vi "Teleop.vi"(10 "Match Info":T2={"Autonomous Elapsed Seconds"=0.0, "TeleOp Elapsed Seconds"=0.0, "Disabled Elapsed Seconds"=0.0, "Visited Autonomous"=FALSE, "Visited TeleOp"=FALSE, "Visited Disabled"=FALSE, "Autonomous Settings"={"Autonomous Style"=enum."Independent", "VI Refnum"=refnum}}, 11 "Call Context":T3) -> ()   [LabVIEW 2015]
doc: "This VI is called for each TeleOp packet received from the DS where the robot is not disabled. It is often used to read from the joysticks and update I/O or to update setpoints for timed control loops. It should complete and return within 20 milliseconds or it may miss DS packets."
uses:
  <vilib>/Rock Robotics/WPI/DriverStation/WPI_DriverStationDerivedRobotMode.ctl
  <vilib>/Rock Robotics/WPI/DriverStation/WPI_DriverStationMatch Info.ctl
  <vilib>/Rock Robotics/SystemInterfaces/spilib/spi_bus.ctl
  <vilib>/Rock Robotics/WPI/CAN/TalonSRX/WPI_CANTalonSRX_APIFeedbackSelect.ctl
  <vilib>/Rock Robotics/WPI/CAN/TalonSRX/WPI_CANTalonSRX_APIControlMode.ctl
  <vilib>/Rock Robotics/WPI/Utilities/WPI_GetSetVariantRefNum.vi
  <vilib>/Rock Robotics/Network Tables/NT Write Boolean Array.vi
  <vilib>/Rock Robotics/Network Tables/NT Write Numeric Array.vi
  <vilib>/Rock Robotics/Network Tables/NT Read Boolean.vi
  <vilib>/Rock Robotics/Network Tables/NT Read Number.vi
  <vilib>/Rock Robotics/WPI/RobotDrive/WPI_RobotDriveArcadeDrive_Standard(NoSaturation).vi
  <vilib>/Rock Robotics/WPI/CAN/Jaguar/SubVIs/WPI_CANJaguar_ControlMode.ctl
  Program Files/National Instruments/LabVIEW 2016/LabVIEW 2016/Targets/NI/RT/VxWorks/vi.lib/Rock Robotics/WPI/CAN/Jaguar/SubVIs/WPI_CANJaguar_SpeedReference.ctl
  <vilib>/Rock Robotics/WPI/Gyro/WPI_GyroAnalogOpen.vi
  <vilib>/Rock Robotics/WPI/MotorControl/WPI_MotorControlOpenCANTalonSRX.vi
  <vilib>/Rock Robotics/Network Tables/NT Write Number.vi
  <vilib>/Rock Robotics/WPI/MotorControl/WPI_MotorControlOpenCANJaguar.vi
panel:
  out "Device Found":bool
  in  "SPI Bus":T1
  in  "Sample Rate (ms)":dbl=1.0 min=0.0 max=100.0 step=0.25 format="%#_13g"
  out "Angle":dbl(knob) scale=0.0..360.0
  in  "stop 2":bool
  in  "Reset Angle?":bool
  out "Calibrated?":bool
  out "Sample Slider 0":dbl(slide) scale=0.0..5.0
  out "Sample Boolean 1":bool
  out "Sample Boolean 0":bool
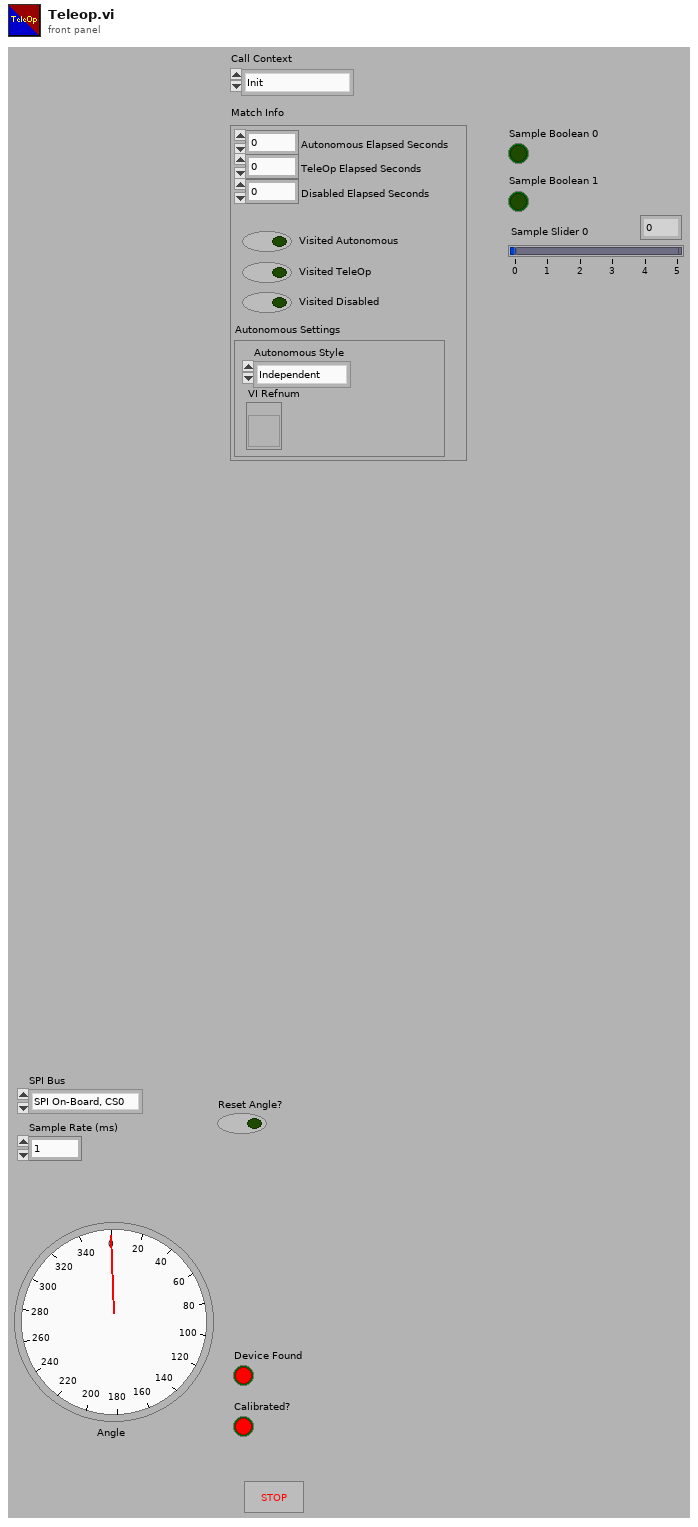
[diagram p1: front panel]
types:
  T1 = typedef "spi_bus.ctl" = enum16{"SPI On-Board, CS0", "SPI On-Board, CS1", "SPI On-Board, CS2", "SPI On-Board, CS3", "SPI MXP", "Invalid"}
  T2 = typedef "WPI_DriverStationMatch Info.ctl" = cluster{"Autonomous Elapsed Seconds":dbl, "TeleOp Elapsed Seconds":dbl, "Disabled Elapsed Seconds":dbl, "Visited Autonomous":bool, "Visited TeleOp":bool, "Visited Disabled":bool, "Autonomous Settings":cluster{"Autonomous Style":enum16{"Iterative", "Independent"}, "VI Refnum":refnum<vi>}}
  T3 = typedef "WPI_DriverStationDerivedRobotMode.ctl" = enum16{"Init", "Execute", "Stop"}
  T4 = typedef "WPI_JoystickDevRef.ctl" = cluster{"Device":T5}
  T5 = typedef "WPI_JoystickDeviceEnum.ctl" = enum16{"USB 0", "USB 1", "USB 2", "USB 3", "USB 4", "USB 5"}
  T6 = cluster{"Axes[0]":dbl, "Axes[1]":dbl, "Axes[2]":dbl, "Axes[3]":dbl, "Axes[4]":dbl, "Axes[5]":dbl, "Axes[6]":dbl, "Axes[7]":dbl, "Axes[8]":dbl}
  T7 = cluster{"Buttons[0]":bool, "Buttons[1]":bool, "Buttons[2]":bool, "Buttons[3]":bool, "Buttons[4]":bool, "Buttons[5]":bool, "Buttons[6]":bool, "Buttons[7]":bool, "Buttons[8]":bool}
  T8 = typedef "WPI_MotorControlDeviceRef.ctl" = cluster{"DeviceStatus":errorcluster, "Type":T9, "PWM":cluster{"PWM Channel":T10, "DeadBand":T11}, "CAN":cluster{"Device Number":u8, "Control Mode":T12, "Semaphore":T13, "Max Vout":dbl, "TalonSRX Control Mode":T14}, "Invert":bool}
  T9 = typedef "WPI_MotorControlType.ctl" = enum16{"PWM", "CAN", "CANTalonSRX"}
  T10 = typedef "FPGA_DIOPWMChannel.ctl" = enum8{"PWM 0", "PWM 1", "PWM 2", "PWM 3", "PWM 4", "PWM 5", "PWM 6", "PWM 7", "PWM 8", "PWM 9", "PWM MXP 0", "PWM MXP 1", "PWM MXP 2", "PWM MXP 3", "PWM MXP 4", "PWM MXP 5", "PWM MXP 6", "PWM MXP 7", "PWM MXP 8", "PWM MXP 9", "Invalid"}
  T11 = typedef "WPI_PWMDeadband.ctl" = cluster{"Name":string, "maxPositivePwm":i32, "minPositivePwm":i32, "centerPwm":i32, "maxNegativePwm":i32, "minNegativePwm":i32, "angularRange":u16}
  T12 = typedef "WPI_CANJaguar_ControlMode.ctl" = enum8{"Percent VBus", "Current", "Speed", "Position", "Voltage"}
  T13 = typedef "Semaphore RefNum" = refnum<k1>
  T14 = typedef "WPI_CANTalonSRX_APIControlMode.ctl" = enum8{"Percent VBus", "Speed", "Position", "Slave", "Unchanged / Invalid", "Voltage Compensation", "Current", "Motion Profile"}
  T15 = typedef "WPI_RobotDriveDevRef.ctl" = cluster{"DevStatus":errorcluster, "Motors[]":T8[], "Square Inputs":bool, "Max Output":dbl}
  T16 = typedef "WPI_SwitchDevRef.ctl" = cluster{"DevStatus":errorcluster, "DIO Channel":T17, "CntIndex":T18, "Normally Closed":bool}
  T17 = typedef "FPGA_DIOChannel.ctl" = enum8{"DIO 0", "DIO 1", "DIO 2", "DIO 3", "DIO 4", "DIO 5", "DIO 6", "DIO 7", "DIO 8", "DIO 9", "DIO MXP 0", "DIO MXP 1", "DIO MXP 2", "DIO MXP 3", "DIO MXP 4", "DIO MXP 5", "DIO MXP 6", "DIO MXP 7", "DIO MXP 8", "DIO MXP 9", "DIO MXP 10", "DIO MXP 11", "DIO MXP 12", "DIO MXP 13", "DIO MXP 14", "DIO MXP 15", "Invalid"}
  T18 = typedef "FPGA_CounterCtrSystemIndex.ctl" = enum8{"Ctr 0", "Ctr 1", "Ctr 2", "Ctr 3", "Ctr 4", "Ctr 5", "Ctr 6", "Ctr 7", "Invalid"}
  T19 = typedef "WPI_GyroDevRef.ctl" = cluster{"DevStatus":errorcluster, "Analog Channel":T20, "Offset":dbl, "Gain (VoltsPerDegree/Second)":dbl, "Gyro Type":enum16{"Analog", "XRS450"}, "Handle":i32, "SPI Bus":T1, "Device Found":bool, "Sample Rate":dbl, "Calibrate On Open":bool}
  T20 = typedef "FPGA_AIChannel.ctl" = enum8{"AI 0", "AI 1", "AI 2", "AI 3", "AI MXP 0", "AI MXP 1", "AI MXP 2", "AI MXP 3", "Invalid"}
  T21 = typedef "WPI_CANTalonSRX_APIFeedbackSelect.ctl" = enum16{"Digital Quadrature Encoder", "Analog Potentiometer", "Analog Encoder", "Count on Quad-A (Rising-Edge)", "Count on Quad-A (Falling-Edge)", "CTR Magnetic Enc (Absolute)", "CTR Magnetic Enc (Relative)", "Pulse Width"}
  T22 = typedef "WPI_CANJaguar_SpeedReference.ctl" = u8
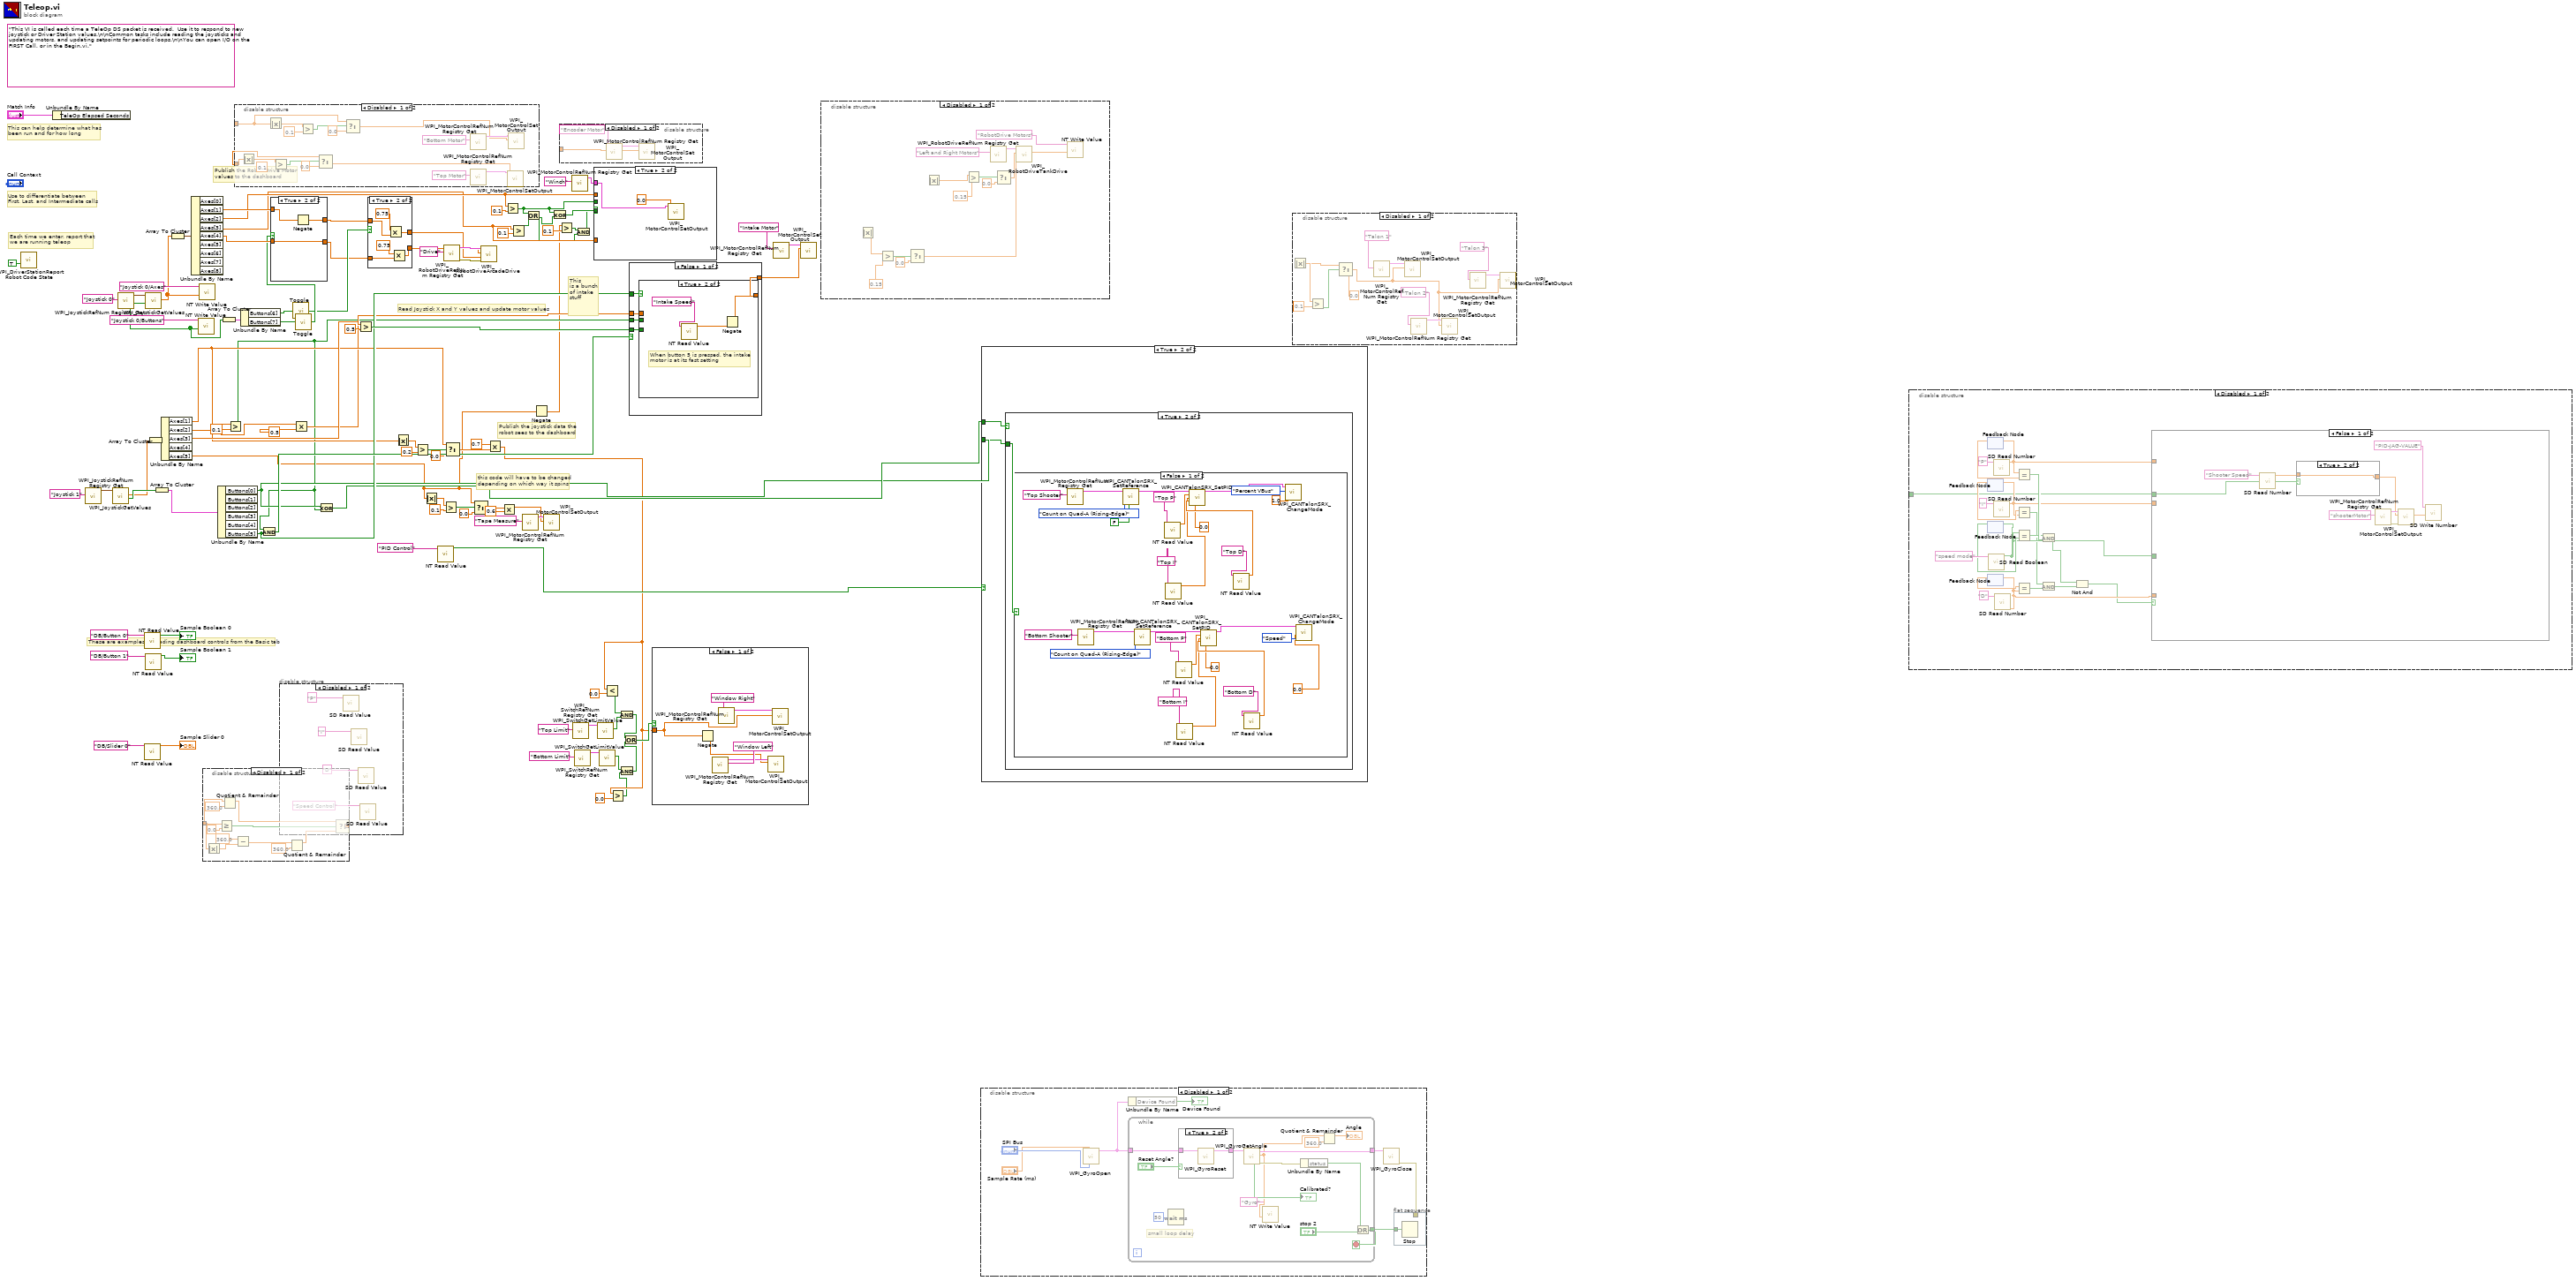
[diagram p0: block diagram]
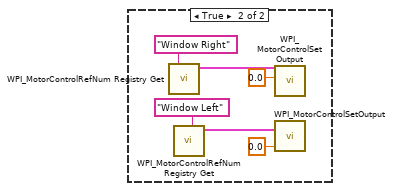
[diagram p2: hidden frame]
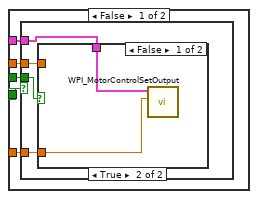
[diagram p3: hidden frame]
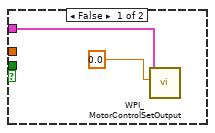
[diagram p4: hidden frame]
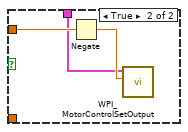
[diagram p5: hidden frame]
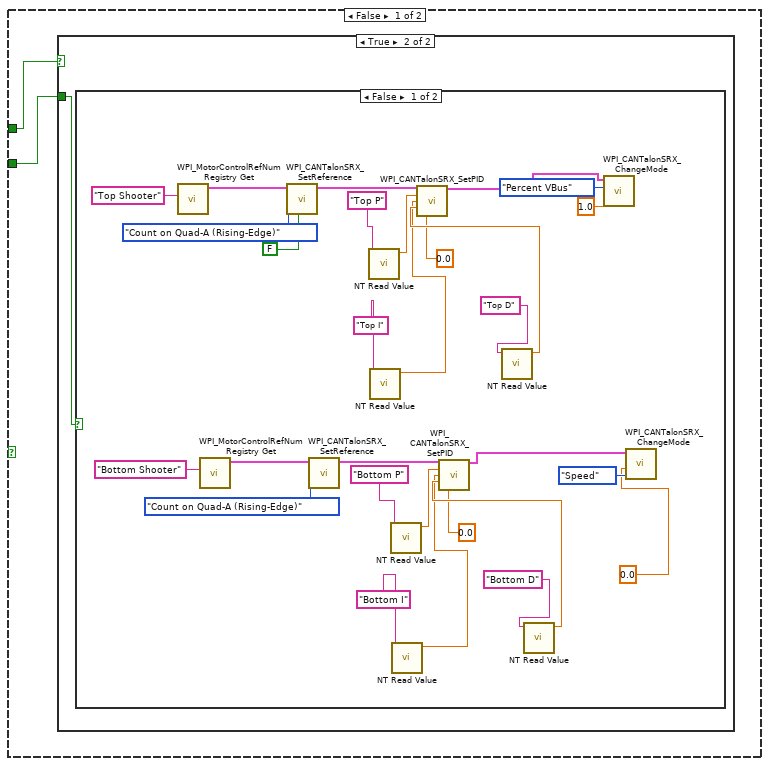
[diagram p6: hidden frame]
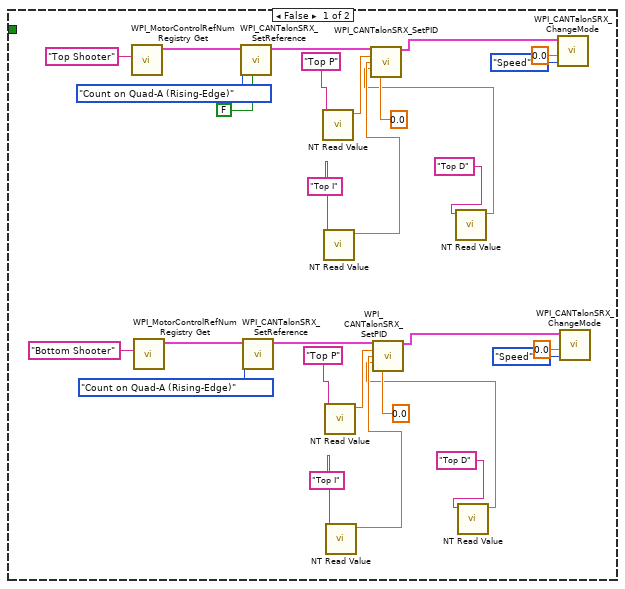
[diagram p7: hidden frame]
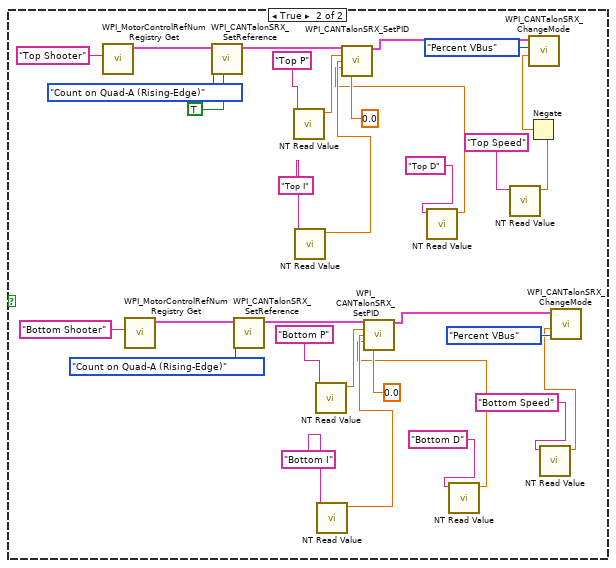
[diagram p8: hidden frame]
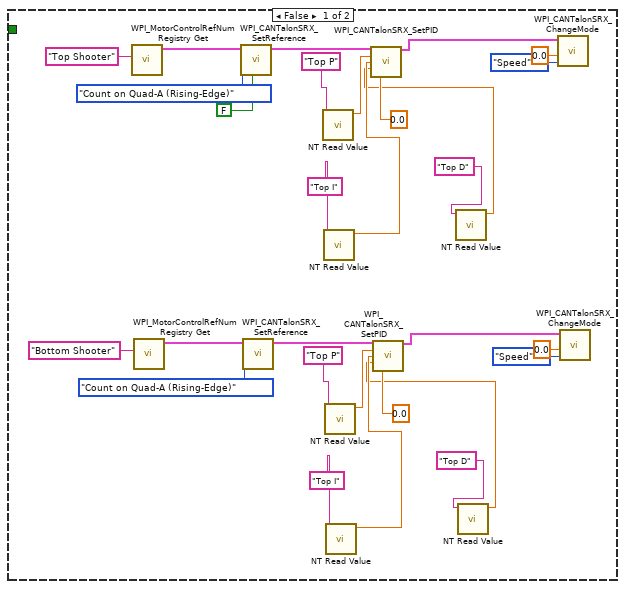
[diagram p9: hidden frame]
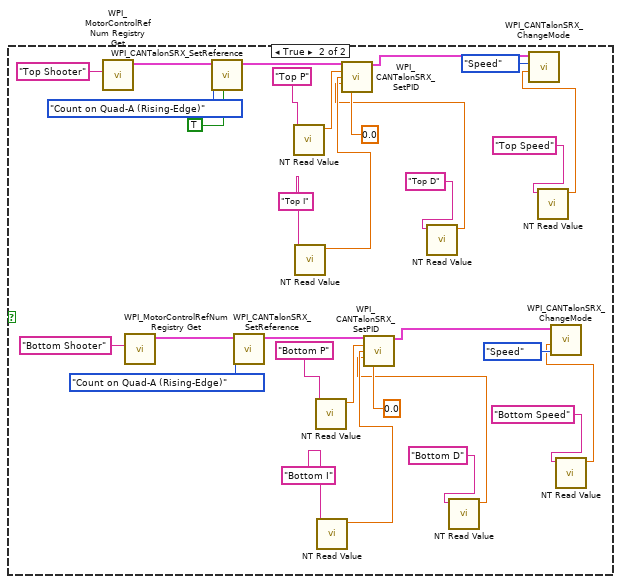
[diagram p10: hidden frame]
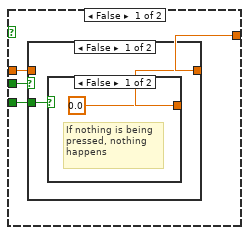
[diagram p14: hidden frame]
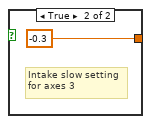
[diagram p15: hidden frame]
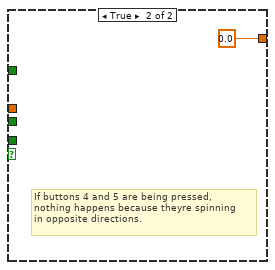
[diagram p17: hidden frame]
diagram:
  (unwired) "This VI is called each time a TeleOp DS packet is received.  Use it to respond to new joystick or Driver Station values.\n\nCommon tasks include reading the joysticks and updating motors, and updating setpoints for periodic loops.\n\nYou can open I/O on the FIRST Call, or in the Begin.vi."
  # "this code will have to be changed\ndepending on which way it spins"
  # "This \nis a bunch\nof intake\nstuff"
  # "These are examples of reading dashboard controls from the Basic tab"
  # "Publish the Robot Drive Motor\nvalues to the dashboard"
  # "Publish the joystick data the\nrobot sees to the dashboard"
  # "Each time we enter, report that\nwe are running teleop"
  # "Use to differentiate between\nFirst, Last, and Intermediate calls"
  # "This can help determine what has\nbeen run and for how long"
  # "Read Joystick X and Y values and update motor values"
  n1 = call <vilib>:"WPI_DriverStationReport Robot Code State.vi"("TeleOp"=TRUE ("Autonomous")) -> ()  [unwired: 10 in, 1 out]
  n2 = Unbundle By Name("Match Info") -> ()  [unwired: 1 out]
  n3 = call <vilib>:"WPI_JoystickRefNum Registry Get.vi"("refnum name"="Joystick 1") -> ("JoystickDevRef"=w75:T4)  [unwired: 1 in, 9 out]
  n4 = call <vilib>:"WPI_JoystickGetValues.vi"("JoystickDevRef"=w75) -> ("Buttons"=w74:bool[], "Axes"=w72:dbl[])  [unwired: 6 in, 3 out]
  n5 = call <vilib>:"WPI_JoystickRefNum Registry Get.vi"("refnum name"="Joystick 0") -> ("JoystickDevRef"=w95:T4)  [unwired: 1 in, 9 out]
  n6 = call-poly <vilib>:"NT Read Value.vi"("Name"="DB/Button 0" ("refnum name")) -> ("Boolean"=→"Sample Boolean 0":bool)  [unwired: 9 in, 1 out]
  n7 = call-poly <vilib>:"NT Read Value.vi"("Name"="DB/Slider 0" ("refnum name")) -> ("Numeric"=→"Sample Slider 0":dbl)  [unwired: 9 in, 1 out]
  n8 = call-poly <vilib>:"NT Read Value.vi"("Name"="DB/Button 1" ("refnum name")) -> ("Boolean"=→"Sample Boolean 1":bool)  [unwired: 9 in, 1 out]
  n9 = call <vilib>:"WPI_JoystickGetValues.vi"("JoystickDevRef"=w95) -> ("Buttons"=w69:bool[], "Axes"=w85:dbl[])  [unwired: 6 in, 3 out]
  n10 = Array To Cluster(array=w72) -> (cluster=w71:T6)
  n11 = Array To Cluster(array=w74) -> (cluster=w73:T7)
  n12 = Unbundle By Name(w71) -> ("Axes[1]"=w56:dbl, "Axes[2]"=w45:dbl, "Axes[3]"=w70:dbl, "Axes[5]"=w27:dbl)  [unwired: 1 out]
  n13 = Array To Cluster(array=w85) -> (cluster=w84:T6)
  n14 = Unbundle By Name(w84) -> ("Axes[1]"=w62:dbl, "Axes[2]"=w30:dbl, "Axes[3]"=w29:dbl, "Axes[4]"=w63:dbl)  [unwired: 5 out]
  n15 = call-poly <vilib>:"NT Write Value.vi"("Boolean Array"=w69, "Name"="Joystick 0/Buttons") -> ()  [unwired: 9 in, 1 out]
  n16 = call-poly <vilib>:"NT Write Value.vi"("Numeric Array"=w85, "Name"="Joystick 0/Axes") -> ()  [unwired: 9 in, 1 out]
  n17 = disable-structure shown="Disabled" {
    disable-tunnel: _ -> [w103 _]
    disable-tunnel: [w98 _] -> _
    frame Disabled {
      n18 = Absolute Value(x=w103) -> (abs(x)=w102:dbl)
      n19 = Greater Or Equal?(x=w103, y=0.0) -> (x >= y?=w106:bool)
      n20 = Quotient & Remainder(x=w103, y=360.0) -> (x-y*floor(x/y)=w105:dbl)  [unwired: 1 out]
      n21 = Subtract(x=360.0, y=w102) -> (x-y=w101:dbl)
      n22 = Quotient & Remainder(x=w101, y=360.0) -> (x-y*floor(x/y)=w99:dbl)  [unwired: 1 out]
      n23 = Select(t=w105, s=w106, f=w99) -> (s? t:f=w98:dbl)
    }
    frame Enabled {
    }
  }
  n24 = Unbundle By Name(w73) -> ("Buttons[0]"=w35:bool, "Buttons[5]"=w77:bool)  [unwired: 4 out]
  n25 = Array To Cluster(array=w69) -> (cluster=w68:T7)
  n26 = Greater?(x=w45, y=0.1) -> (0:w34:bool)
  n27 = disable-structure shown="Disabled" {
    disable-tunnel: _ -> [w116 _]
    disable-tunnel: _ -> [w109 _]
    frame Disabled {
      n28 = Absolute Value(x=w116) -> (abs(x)=w119:dbl)
      n29 = Absolute Value(x=w109) -> (abs(x)=w114:dbl)
      n30 = Greater?(x=w119, y=0.1) -> (0:w117:bool)
      n31 = Greater?(x=w114, y=0.1) -> (0:w112:bool)
      n32 = Select(t=w116, s=w117, f=0.0) -> (s? t:f=w120:dbl)
      n33 = Select(t=w109, s=w112, f=0.0) -> (s? t:f=w110:dbl)
      n34 = call <vilib>:"WPI_MotorControlRefNum Registry Get.vi"("refnum name"="Bottom Motor") -> ("MotorControlDevRef"=w121:T8)  [unwired: 9 in, 1 out]
      n35 = call <vilib>:"WPI_MotorControlRefNum Registry Get.vi"("refnum name"="Top Motor") -> ("MotorControlDevRef"=w122:T8)  [unwired: 9 in, 1 out]
      n36 = call <vilib>:"WPI_MotorControlSetOutput.vi"("Output"=w120, "MotorControlDevRef"=w122) -> ()  [unwired: 7 in, 3 out]
      n37 = call <vilib>:"WPI_MotorControlSetOutput.vi"("Output"=w110, "MotorControlDevRef"=w121) -> ()  [unwired: 7 in, 3 out]
    }
    frame Enabled {
    }
  }
  n38 = Unbundle By Name(w68) -> ("Buttons[6]"=w53:bool, "Buttons[7]"=w67:bool)
  n39 = And(x=w34, y=w77) -> (x .and. y?=w81:bool)
  n40 = disable-structure shown="Disabled" {
    frame Disabled {
      n41 = call-poly <vilib>:"SD Read Value.vi"("Name"="P") -> ()  [unwired: 8 in, 3 out]
      n42 = call-poly <vilib>:"SD Read Value.vi"("Name"="I") -> ()  [unwired: 8 in, 3 out]
      n43 = call-poly <vilib>:"SD Read Value.vi"("Name"="D") -> ()  [unwired: 8 in, 3 out]
      n44 = call-poly <vilib>:"SD Read Value.vi"("Name"="Speed Control") -> ()  [unwired: 8 in, 3 out]
    }
    frame Enabled {
    }
  }
  n45 = call "Toggle.vi"("Input"=w53) -> ("Output"=w52:bool)
  n46 = Multiply(x=w45, y=0.5) -> (x*y=w47:dbl)
  n47 = call "Toggle.vi"("Input"=w67) -> ("Output"=w61:bool)
  n48 = case shown="True" w61 {
    tunnel: [w129 w133] -> w51
    tunnel: w63 -> [w129 w133]
    tunnel: [w130 w131] -> w50
    tunnel: w62 -> [w130 w132]
    frame False {
    }
    frame True {
      n49 = Negate(x=w132) -> (-x=w131:dbl)
    }
  }
  n50 = Exclusive Or(1:w34, 2:w35) -> (0:w36:bool)
  n51 = Greater?(x=w70, y=0.5) -> (0:w79:bool)
  n52 = case shown="True" w52 {
    tunnel: w51 -> [w134 w139]
    tunnel: w50 -> [w135 w138]
    tunnel: [w135 w137] -> w49
    tunnel: [w134 w136] -> w48
    frame False {
    }
    frame True {
      n53 = Multiply(x=0.75, y=w138) -> (x*y=w137:dbl)
      n54 = Multiply(x=0.75, y=w139) -> (x*y=w136:dbl)
    }
  }
  n55 = Absolute Value(x=w56) -> (abs(x)=w57:dbl)
  n56 = Greater?(x=w57, y=0.2) -> (0:w59:bool)
  n57 = Absolute Value(x=w27) -> (abs(x)=w41:dbl)
  n58 = call-poly <vilib>:"NT Read Value.vi"("Name"="PID Control") -> ("Boolean"=w15:bool)  [unwired: 9 in, 1 out]
  n59 = Greater?(x=w41, y=0.1) -> (0:w43:bool)
  n60 = call <vilib>:"WPI_RobotDriveRefNum Registry Get.vi"("refnum name"="Drive") -> ("error out"=w64:errorcluster, "RobotDriveDevRef"=w65:T15)  [unwired: 1 in, 8 out]
  n61 = Select(t=w56, s=w59, f=0.0) -> (s? t:f=w60:dbl)
  n62 = Select(t=w27, s=w43, f=0.0) -> (s? t:f=w37:dbl)
  n63 = call-poly <vilib>:"WPI_RobotDriveArcadeDrive.vi"("error in (no error)"=w64, "Y axis value"=w49, "X axis value"=w48, "RobotDriveDevRef"=w65) -> ()  [unwired: 5 in, 3 out]
  n64 = Multiply(x=0.7, y=w60) -> (x*y=w7:dbl)
  n65 = Multiply(x=w37, y=0.6) -> (x*y=w22:dbl)
  n66 = Greater?(x=w30, y=0.1) -> (0:w25:bool)
  n67 = Greater?(x=w29, y=0.1) -> (0:w24:bool)
  n68 = call <vilib>:"WPI_MotorControlRefNum Registry Get.vi"("refnum name"="Tape Measure") -> ("MotorControlDevRef"=w39:T8)  [unwired: 9 in, 1 out]
  n69 = Or(x=w25, y=w24) -> (x .or. y?=w23:bool)
  n70 = Negate(x=w27) -> (-x=w17:dbl)
  n71 = call <vilib>:"WPI_MotorControlSetOutput.vi"("Output"=w22, "MotorControlDevRef"=w39) -> ()  [unwired: 7 in, 3 out]
  n72 = Exclusive Or(1:w24, 2:w25) -> (0:w31:bool)
  n73 = Greater?(x=w17, y=0.1) -> (0:w26:bool)
  n74 = disable-structure shown="Disabled" {
    disable-tunnel: _ -> [w142 _]
    frame Disabled {
      n75 = call <vilib>:"WPI_MotorControlRefNum Registry Get.vi"("refnum name"="Encoder Motor") -> ("MotorControlDevRef"=w143:T8)  [unwired: 9 in, 1 out]
      n76 = call <vilib>:"WPI_MotorControlSetOutput.vi"("Output"=w142, "MotorControlDevRef"=w143) -> ()  [unwired: 7 in, 3 out]
    }
    frame Enabled {
    }
  }
  n77 = call <vilib>:"WPI_MotorControlRefNum Registry Get.vi"("refnum name"="Winch") -> ("MotorControlDevRef"=w18:T8)  [unwired: 9 in, 1 out]
  n78 = call <vilib>:"WPI_SwitchRefNum Registry Get.vi"("refnum name"="Top Limit") -> ("SwitchDevRef"=w14:T16)  [unwired: 9 in, 1 out]
  n79 = call <vilib>:"WPI_SwitchRefNum Registry Get.vi"("refnum name"="Bottom Limit") -> ("SwitchDevRef"=w12:T16)  [unwired: 9 in, 1 out]
  n80 = And(x=w26, y=w23) -> (x .and. y?=w20:bool)
  n81 = case shown="True" w20 {
    tunnel: w31 -> [w149 _]
    tunnel: w30 -> [w148 _]
    tunnel: w29 -> [w147 _]
    tunnel: w25 -> [w146 _]
    tunnel: w18 -> [w145 w161]
    frame False {
      n82 = case shown="True" w149 {
        tunnel: w146 -> [_ w155]
        tunnel: w148 -> [_ w154]
        tunnel: w147 -> [_ w153]
        tunnel: w145 -> [w150 w152]
        frame False {
          n83 = call <vilib>:"WPI_MotorControlSetOutput.vi"("Output"=0.0, "MotorControlDevRef"=w150) -> ()  [unwired: 7 in, 3 out]
        }
        frame True {
          n84 = case shown="False" w155 {
            tunnel: w154 -> [_ w160]
            tunnel: w153 -> [w157 _]
            tunnel: w152 -> [w156 w158]
            frame False {
              n85 = call <vilib>:"WPI_MotorControlSetOutput.vi"("Output"=w157, "MotorControlDevRef"=w156) -> ()  [unwired: 7 in, 3 out]
            }
            frame True {
              n86 = Negate(x=w160) -> (-x=w159:dbl)
              n87 = call <vilib>:"WPI_MotorControlSetOutput.vi"("Output"=w159, "MotorControlDevRef"=w158) -> ()  [unwired: 7 in, 3 out]
            }
          }
        }
      }
    }
    frame True {
      n88 = call <vilib>:"WPI_MotorControlSetOutput.vi"("Output"=0.0, "MotorControlDevRef"=w161) -> ()  [unwired: 7 in, 3 out]
    }
  }
  n89 = call <vilib>:"WPI_SwitchGetLimitValue.vi"("SwitchDevRef"=w14) -> ("Switch Pressed"=w1:bool)  [unwired: 8 in, 2 out]
  n90 = call <vilib>:"WPI_SwitchGetLimitValue.vi"("SwitchDevRef"=w12) -> ("Switch Pressed"=w5:bool)  [unwired: 8 in, 2 out]
  n91 = Less?(x=w7, y=0.0) -> (x < y?=w8:bool)
  n92 = Greater?(x=w7, y=0.0) -> (0:w4:bool)
  n93 = And(x=w8, y=w1) -> (x .and. y?=w2:bool)
  n94 = And(x=w5, y=w4) -> (x .and. y?=w3:bool)
  n95 = Or(x=w2, y=w3) -> (x .or. y?=w10:bool)
  n96 = case shown="False" w81 {
    tunnel: [w166 0.0] -> w78
    tunnel: w77 -> [w167 _]
    tunnel: w79 -> [w165 _]
    tunnel: w47 -> [w164 _]
    tunnel: w34 -> [w163 _]
    frame False {
      n97 = case shown="True" w167 {
        tunnel: [w171 w177] -> w166
        tunnel: w165 -> [w170 _]
        tunnel: w164 -> [w169 _]
        tunnel: w163 -> [w168 _]
        frame False {
          n98 = case shown="False" w168 {
            tunnel: [w172 w176] -> w171
            tunnel: w170 -> [w173 _]
            tunnel: w169 -> [_ w176]
            frame False {
              n99 = case shown="False" w173 {
                tunnel: [0.0 -0.3] -> w172
                frame False {
                  # "If nothing is being\npressed, nothing \nhappens"
                }
                frame True {
                  # "Intake slow setting\nfor axes 3"
                }
              }
            }
            frame True {
              # "When button\n4 is being pressed,\nthe outake is activated"
            }
          }
        }
        frame True {
          # "When button 5 is pressed, the intake \nmotor is at its fast setting"
          n100 = call-poly <vilib>:"NT Read Value.vi"("Name"="Intake Speed") -> ("Numeric"=w178:dbl)  [unwired: 9 in, 1 out]
          n101 = Negate(x=w178) -> (-x=w177:dbl)
        }
      }
    }
    frame True {
      # "If buttons 4 and 5 are being pressed,\nnothing happens because theyre spinning\nin opposite directions."
    }
  }
  n102 = case shown="False" w10 {
    tunnel: w7 -> [w181 _]
    frame False {
      n103 = Negate(x=w181) -> (-x=w182:dbl)
      n104 = call <vilib>:"WPI_MotorControlRefNum Registry Get.vi"("refnum name"="Window Left") -> ("MotorControlDevRef"=w185:T8)  [unwired: 9 in, 1 out]
      n105 = call <vilib>:"WPI_MotorControlRefNum Registry Get.vi"("refnum name"="Window Right") -> ("MotorControlDevRef"=w184:T8)  [unwired: 9 in, 1 out]
      n106 = call <vilib>:"WPI_MotorControlSetOutput.vi"("Output"=w182, "MotorControlDevRef"=w185) -> ()  [unwired: 7 in, 3 out]
      n107 = call <vilib>:"WPI_MotorControlSetOutput.vi"("Output"=w181, "MotorControlDevRef"=w184) -> ()  [unwired: 7 in, 3 out]
    }
    frame True {
      n108 = call <vilib>:"WPI_MotorControlRefNum Registry Get.vi"("refnum name"="Window Right") -> ("MotorControlDevRef"=w191:T8)  [unwired: 9 in, 1 out]
      n109 = call <vilib>:"WPI_MotorControlRefNum Registry Get.vi"("refnum name"="Window Left") -> ("MotorControlDevRef"=w190:T8)  [unwired: 9 in, 1 out]
      n110 = call <vilib>:"WPI_MotorControlSetOutput.vi"("Output"=0.0, "MotorControlDevRef"=w191) -> ()  [unwired: 7 in, 3 out]
      n111 = call <vilib>:"WPI_MotorControlSetOutput.vi"("Output"=0.0, "MotorControlDevRef"=w190) -> ()  [unwired: 7 in, 3 out]
    }
  }
  n112 = call <vilib>:"WPI_MotorControlRefNum Registry Get.vi"("refnum name"="Intake Motor") -> ("MotorControlDevRef"=w82:T8)  [unwired: 9 in, 1 out]
  n113 = call <vilib>:"WPI_MotorControlSetOutput.vi"("Output"=w78, "MotorControlDevRef"=w82) -> ()  [unwired: 7 in, 3 out]
  n114 = disable-structure shown="Disabled" {
    frame Disabled {
      n115 = Absolute Value() -> (abs(x)=w194:dbl)  [unwired: 1 in]
      n116 = Greater?(x=w194, y=0.15 ("x")) -> (0:w199:bool)
      n117 = Select(s=w199, f=0.0) -> (s? t:f=w197:dbl)  [unwired: 1 in]
      n118 = Absolute Value() -> (abs(x)=w193:dbl)  [unwired: 1 in]
      n119 = Greater?(x=w193, y=0.15 ("x")) -> (0:w202:bool)
      n120 = call <vilib>:"WPI_RobotDriveRefNum Registry Get.vi"("refnum name"="Left and Right Motors") -> ("RobotDriveDevRef"=w205:T15)  [unwired: 1 in, 9 out]
      n121 = Select(s=w202, f=0.0) -> (s? t:f=w200:dbl)  [unwired: 1 in]
      n122 = call <vilib>:"WPI_RobotDriveTankDrive.vi"("Right axis value"=w197, "Left axis value"=w200, "RobotDriveDevRef"=w205) -> ("Motor Values"=w204:dbl[])  [unwired: 6 in, 2 out]
      n123 = call-poly <vilib>:"NT Write Value.vi"("Numeric Array"=w204, "Name"="RobotDrive Motors") -> ()  [unwired: 9 in, 1 out]
    }
    frame Enabled {
    }
  }
  n124 = disable-structure shown="Disabled" {
    frame Disabled {
      n125 = call-poly <vilib>:"WPI_GyroOpen.vi"("Calibrated Center Voltage"="SPI Bus", "Calibration Time (s)"="Sample Rate (ms)") -> ("GyroDevRef"=w209:T19)  [unwired: 7 in, 2 out]
      n126 = Unbundle By Name(w209) -> ("Device Found"=→"Device Found":bool)
      n127 = while {
        tunnel: w209 -> [w224]
        tunnel: [w221] -> w211
        tunnel: [w219] -> w212
        stop <- w221 stop-if-true
        # "small loop delay"
        n128 = Wait (ms)(milliseconds to wait=u32 50) -> ()  [unwired: 1 out]
        n129 = case shown="True" "Reset Angle?" {
          tunnel: w224 -> [w229 w231]
          tunnel: [w229 w230] -> w220
          frame False {
          }
          frame True {
            n130 = call <vilib>:"WPI_GyroReset.vi"("GyroDevRef"=w231) -> ("GyroDevRef"=w230:T19)  [unwired: 9 in, 1 out]
          }
        }
        n131 = call <vilib>:"WPI_GyroGetAngle.vi"("GyroDevRef"=w220) -> ("error out"=w218:errorcluster, "Angle"=w216:dbl, "GyroDevRef"=w219:T19, "Calibrated?"=→"Calibrated?":bool)  [unwired: 6 in, 1 out]
        n132 = call-poly <vilib>:"NT Write Value.vi"("Numeric"=w216, "Name"="Gyro") -> ()  [unwired: 9 in, 1 out]
        n133 = Unbundle By Name(w218) -> ("status"=w222:bool)
        n134 = Quotient & Remainder(x=w216, y=360.0) -> (x-y*floor(x/y)=→"Angle":dbl)  [unwired: 1 out]
        n135 = Or(x=w222, y="stop 2") -> (x .or. y?=w221:bool)
      }
      n136 = call <vilib>:"WPI_GyroClose.vi"("GyroDevRef"=w212) -> ("error out"=w210:errorcluster)  [unwired: 10 in]
      n137 = flat-sequence {
        tunnel: w211 -> [w214]
        tunnel: w210 -> [_]
        frame #0 {
          n138 = Stop(stop? (T)=w214) -> ()
        }
      }
    }
    frame Enabled {
    }
  }
  n139 = case shown="True" w15 {
    tunnel: w36 -> [w233 w326]
    tunnel: w35 -> [w232 w325]
    frame False {
      n140 = case shown="True" w233 {
        tunnel: w232 -> [_ w263]
        frame False {
          n141 = call <vilib>:"WPI_MotorControlRefNum Registry Get.vi"("refnum name"="Top Shooter") -> ("MotorControlDevRef"=w261:T8)  [unwired: 9 in, 1 out]
          n142 = call <vilib>:"WPI_MotorControlRefNum Registry Get.vi"("refnum name"="Bottom Shooter") -> ("MotorControlDevRef"=w247:T8)  [unwired: 9 in, 1 out]
          n143 = call <vilib>:"WPI_CANTalonSRX_SetReference.vi"("Reverse Closed-Loop Output"=FALSE, "Feedback Reference"=WPI_CANTalonSRX_APIFeedbackSelect."Count on Quad-A (Rising-Edge)", "CAN Talon SRX Ref"=w261) -> ("CAN Talon SRX Ref"=w262:T8)  [unwired: 7 in, 1 out]
          n144 = call <vilib>:"WPI_CANTalonSRX_SetReference.vi"("Feedback Reference"=WPI_CANTalonSRX_APIFeedbackSelect."Count on Quad-A (Rising-Edge)", "CAN Talon SRX Ref"=w247) -> ("CAN Talon SRX Ref"=w248:T8)  [unwired: 8 in, 1 out]
          n145 = call-poly <vilib>:"NT Read Value.vi"("Name"="Top P") -> ("Numeric"=w252:dbl)  [unwired: 9 in, 1 out]
          n146 = call-poly <vilib>:"NT Read Value.vi"("Name"="Top I") -> ("Numeric"=w251:dbl)  [unwired: 9 in, 1 out]
          n147 = call-poly <vilib>:"NT Read Value.vi"("Name"="Top P") -> ("Numeric"=w238:dbl)  [unwired: 9 in, 1 out]
          n148 = call-poly <vilib>:"NT Read Value.vi"("Name"="Top I") -> ("Numeric"=w237:dbl)  [unwired: 9 in, 1 out]
          n149 = call-poly <vilib>:"NT Read Value.vi"("Name"="Top D") -> ("Numeric"=w250:dbl)  [unwired: 9 in, 1 out]
          n150 = call <vilib>:"WPI_CANTalonSRX_SetPID.vi"("CAN Talon SRX Ref"=w262, "P"=w252, "I"=w251, "D"=w250, "F"=0.0) -> ("CAN Talon SRX Ref"=w258:T8)  [unwired: 9 in, 1 out]
          n151 = call-poly <vilib>:"NT Read Value.vi"("Name"="Top D") -> ("Numeric"=w236:dbl)  [unwired: 9 in, 1 out]
          n152 = call <vilib>:"WPI_CANTalonSRX_SetPID.vi"("CAN Talon SRX Ref"=w248, "P"=w238, "I"=w237, "D"=w236, "F"=0.0) -> ("CAN Talon SRX Ref"=w244:T8)  [unwired: 9 in, 1 out]
          n153 = call <vilib>:"WPI_CANTalonSRX_ChangeMode.vi"("Output"=0.0, "Control Mode"=WPI_CANTalonSRX_APIControlMode."Speed", "CAN Talon SRX Ref"=w258) -> ()  [unwired: 7 in, 2 out]
          n154 = call <vilib>:"WPI_CANTalonSRX_ChangeMode.vi"("Output"=0.0, "Control Mode"=WPI_CANTalonSRX_APIControlMode."Speed", "CAN Talon SRX Ref"=w244) -> ()  [unwired: 7 in, 2 out]
        }
        frame True {
          n155 = case shown="False" w263 {
            frame False {
              n156 = call <vilib>:"WPI_MotorControlRefNum Registry Get.vi"("refnum name"="Top Shooter") -> ("MotorControlDevRef"=w268:T8)  [unwired: 9 in, 1 out]
              n157 = call <vilib>:"WPI_MotorControlRefNum Registry Get.vi"("refnum name"="Bottom Shooter") -> ("MotorControlDevRef"=w281:T8)  [unwired: 9 in, 1 out]
              n158 = call <vilib>:"WPI_CANTalonSRX_SetReference.vi"("Reverse Closed-Loop Output"=FALSE, "Feedback Reference"=WPI_CANTalonSRX_APIFeedbackSelect."Count on Quad-A (Rising-Edge)", "CAN Talon SRX Ref"=w268) -> ("CAN Talon SRX Ref"=w267:T8)  [unwired: 7 in, 1 out]
              n159 = call <vilib>:"WPI_CANTalonSRX_SetReference.vi"("Feedback Reference"=WPI_CANTalonSRX_APIFeedbackSelect."Count on Quad-A (Rising-Edge)", "CAN Talon SRX Ref"=w281) -> ("CAN Talon SRX Ref"=w280:T8)  [unwired: 8 in, 1 out]
              n160 = call-poly <vilib>:"NT Read Value.vi"("Name"="Top P") -> ("Numeric"=w275:dbl)  [unwired: 9 in, 1 out]
              n161 = call-poly <vilib>:"NT Read Value.vi"("Name"="Top I") -> ("Numeric"=w276:dbl)  [unwired: 9 in, 1 out]
              n162 = call-poly <vilib>:"NT Read Value.vi"("Name"="Bottom P") -> ("Numeric"=w289:dbl)  [unwired: 9 in, 1 out]
              n163 = call-poly <vilib>:"NT Read Value.vi"("Name"="Bottom I") -> ("Numeric"=w290:dbl)  [unwired: 9 in, 1 out]
              n164 = call-poly <vilib>:"NT Read Value.vi"("Name"="Top D") -> ("Numeric"=w277:dbl)  [unwired: 9 in, 1 out]
              n165 = call <vilib>:"WPI_CANTalonSRX_SetPID.vi"("CAN Talon SRX Ref"=w267, "P"=w275, "I"=w276, "D"=w277, "F"=0.0) -> ("CAN Talon SRX Ref"=w266:T8)  [unwired: 9 in, 1 out]
              n166 = call-poly <vilib>:"NT Read Value.vi"("Name"="Bottom D") -> ("Numeric"=w291:dbl)  [unwired: 9 in, 1 out]
              n167 = call <vilib>:"WPI_CANTalonSRX_SetPID.vi"("CAN Talon SRX Ref"=w280, "P"=w289, "I"=w290, "D"=w291, "F"=0.0) -> ("CAN Talon SRX Ref"=w284:T8)  [unwired: 9 in, 1 out]
              n168 = call <vilib>:"WPI_CANTalonSRX_ChangeMode.vi"("Output"=1.0, "Control Mode"=WPI_CANTalonSRX_APIControlMode."Percent VBus", "CAN Talon SRX Ref"=w266) -> ()  [unwired: 7 in, 2 out]
              n169 = call <vilib>:"WPI_CANTalonSRX_ChangeMode.vi"("Output"=0.0, "Control Mode"=WPI_CANTalonSRX_APIControlMode."Speed", "CAN Talon SRX Ref"=w284) -> ()  [unwired: 7 in, 2 out]
            }
            frame True {
              n170 = call <vilib>:"WPI_MotorControlRefNum Registry Get.vi"("refnum name"="Top Shooter") -> ("MotorControlDevRef"=w323:T8)  [unwired: 9 in, 1 out]
              n171 = call <vilib>:"WPI_MotorControlRefNum Registry Get.vi"("refnum name"="Bottom Shooter") -> ("MotorControlDevRef"=w309:T8)  [unwired: 9 in, 1 out]
              n172 = call <vilib>:"WPI_CANTalonSRX_SetReference.vi"("Reverse Closed-Loop Output"=TRUE, "Feedback Reference"=WPI_CANTalonSRX_APIFeedbackSelect."Count on Quad-A (Rising-Edge)", "CAN Talon SRX Ref"=w323) -> ("CAN Talon SRX Ref"=w324:T8)  [unwired: 7 in, 1 out]
              n173 = call <vilib>:"WPI_CANTalonSRX_SetReference.vi"("Feedback Reference"=WPI_CANTalonSRX_APIFeedbackSelect."Count on Quad-A (Rising-Edge)", "CAN Talon SRX Ref"=w309) -> ("CAN Talon SRX Ref"=w310:T8)  [unwired: 8 in, 1 out]
              n174 = call-poly <vilib>:"NT Read Value.vi"("Name"="Top P") -> ("Numeric"=w315:dbl)  [unwired: 9 in, 1 out]
              n175 = call-poly <vilib>:"NT Read Value.vi"("Name"="Top I") -> ("Numeric"=w314:dbl)  [unwired: 9 in, 1 out]
              n176 = call-poly <vilib>:"NT Read Value.vi"("Name"="Bottom P") -> ("Numeric"=w301:dbl)  [unwired: 9 in, 1 out]
              n177 = call-poly <vilib>:"NT Read Value.vi"("Name"="Bottom I") -> ("Numeric"=w300:dbl)  [unwired: 9 in, 1 out]
              n178 = call-poly <vilib>:"NT Read Value.vi"("Name"="Top D") -> ("Numeric"=w313:dbl)  [unwired: 9 in, 1 out]
              n179 = call <vilib>:"WPI_CANTalonSRX_SetPID.vi"("CAN Talon SRX Ref"=w324, "P"=w315, "I"=w314, "D"=w313, "F"=0.0) -> ("CAN Talon SRX Ref"=w320:T8)  [unwired: 9 in, 1 out]
              n180 = call-poly <vilib>:"NT Read Value.vi"("Name"="Bottom D") -> ("Numeric"=w299:dbl)  [unwired: 9 in, 1 out]
              n181 = call <vilib>:"WPI_CANTalonSRX_SetPID.vi"("CAN Talon SRX Ref"=w310, "P"=w301, "I"=w300, "D"=w299, "F"=0.0) -> ("CAN Talon SRX Ref"=w306:T8)  [unwired: 9 in, 1 out]
              n182 = call-poly <vilib>:"NT Read Value.vi"("Name"="Top Speed") -> ("Numeric"=w294:dbl)  [unwired: 9 in, 1 out]
              n183 = Negate(x=w294) -> (-x=w293:dbl)
              n184 = call <vilib>:"WPI_CANTalonSRX_ChangeMode.vi"("Output"=w293, "Control Mode"=WPI_CANTalonSRX_APIControlMode."Percent VBus", "CAN Talon SRX Ref"=w320) -> ()  [unwired: 7 in, 2 out]
              n185 = call-poly <vilib>:"NT Read Value.vi"("Name"="Bottom Speed") -> ("Numeric"=w296:dbl)  [unwired: 9 in, 1 out]
              n186 = call <vilib>:"WPI_CANTalonSRX_ChangeMode.vi"("Output"=w296, "Control Mode"=WPI_CANTalonSRX_APIControlMode."Percent VBus", "CAN Talon SRX Ref"=w306) -> ()  [unwired: 7 in, 2 out]
            }
          }
        }
      }
    }
    frame True {
      n187 = case shown="True" w326 {
        tunnel: w325 -> [_ w356]
        frame False {
          n188 = call <vilib>:"WPI_MotorControlRefNum Registry Get.vi"("refnum name"="Top Shooter") -> ("MotorControlDevRef"=w354:T8)  [unwired: 9 in, 1 out]
          n189 = call <vilib>:"WPI_MotorControlRefNum Registry Get.vi"("refnum name"="Bottom Shooter") -> ("MotorControlDevRef"=w340:T8)  [unwired: 9 in, 1 out]
          n190 = call <vilib>:"WPI_CANTalonSRX_SetReference.vi"("Reverse Closed-Loop Output"=FALSE, "Feedback Reference"=WPI_CANTalonSRX_APIFeedbackSelect."Count on Quad-A (Rising-Edge)", "CAN Talon SRX Ref"=w354) -> ("CAN Talon SRX Ref"=w355:T8)  [unwired: 7 in, 1 out]
          n191 = call <vilib>:"WPI_CANTalonSRX_SetReference.vi"("Feedback Reference"=WPI_CANTalonSRX_APIFeedbackSelect."Count on Quad-A (Rising-Edge)", "CAN Talon SRX Ref"=w340) -> ("CAN Talon SRX Ref"=w341:T8)  [unwired: 8 in, 1 out]
          n192 = call-poly <vilib>:"NT Read Value.vi"("Name"="Top P") -> ("Numeric"=w345:dbl)  [unwired: 9 in, 1 out]
          n193 = call-poly <vilib>:"NT Read Value.vi"("Name"="Top I") -> ("Numeric"=w344:dbl)  [unwired: 9 in, 1 out]
          n194 = call-poly <vilib>:"NT Read Value.vi"("Name"="Top P") -> ("Numeric"=w331:dbl)  [unwired: 9 in, 1 out]
          n195 = call-poly <vilib>:"NT Read Value.vi"("Name"="Top I") -> ("Numeric"=w330:dbl)  [unwired: 9 in, 1 out]
          n196 = call-poly <vilib>:"NT Read Value.vi"("Name"="Top D") -> ("Numeric"=w343:dbl)  [unwired: 9 in, 1 out]
          n197 = call <vilib>:"WPI_CANTalonSRX_SetPID.vi"("CAN Talon SRX Ref"=w355, "P"=w345, "I"=w344, "D"=w343, "F"=0.0) -> ("CAN Talon SRX Ref"=w351:T8)  [unwired: 9 in, 1 out]
          n198 = call-poly <vilib>:"NT Read Value.vi"("Name"="Top D") -> ("Numeric"=w329:dbl)  [unwired: 9 in, 1 out]
          n199 = call <vilib>:"WPI_CANTalonSRX_SetPID.vi"("CAN Talon SRX Ref"=w341, "P"=w331, "I"=w330, "D"=w329, "F"=0.0) -> ("CAN Talon SRX Ref"=w337:T8)  [unwired: 9 in, 1 out]
          n200 = call <vilib>:"WPI_CANTalonSRX_ChangeMode.vi"("Output"=0.0, "Control Mode"=WPI_CANTalonSRX_APIControlMode."Speed", "CAN Talon SRX Ref"=w351) -> ()  [unwired: 7 in, 2 out]
          n201 = call <vilib>:"WPI_CANTalonSRX_ChangeMode.vi"("Output"=0.0, "Control Mode"=WPI_CANTalonSRX_APIControlMode."Speed", "CAN Talon SRX Ref"=w337) -> ()  [unwired: 7 in, 2 out]
        }
        frame True {
          n202 = case shown="False" w356 {
            frame False {
              n203 = call <vilib>:"WPI_MotorControlRefNum Registry Get.vi"("refnum name"="Top Shooter") -> ("MotorControlDevRef"=w361:T8)  [unwired: 9 in, 1 out]
              n204 = call <vilib>:"WPI_MotorControlRefNum Registry Get.vi"("refnum name"="Bottom Shooter") -> ("MotorControlDevRef"=w374:T8)  [unwired: 9 in, 1 out]
              n205 = call <vilib>:"WPI_CANTalonSRX_SetReference.vi"("Reverse Closed-Loop Output"=FALSE, "Feedback Reference"=WPI_CANTalonSRX_APIFeedbackSelect."Count on Quad-A (Rising-Edge)", "CAN Talon SRX Ref"=w361) -> ("CAN Talon SRX Ref"=w360:T8)  [unwired: 7 in, 1 out]
              n206 = call <vilib>:"WPI_CANTalonSRX_SetReference.vi"("Feedback Reference"=WPI_CANTalonSRX_APIFeedbackSelect."Count on Quad-A (Rising-Edge)", "CAN Talon SRX Ref"=w374) -> ("CAN Talon SRX Ref"=w373:T8)  [unwired: 8 in, 1 out]
              n207 = call-poly <vilib>:"NT Read Value.vi"("Name"="Top P") -> ("Numeric"=w368:dbl)  [unwired: 9 in, 1 out]
              n208 = call-poly <vilib>:"NT Read Value.vi"("Name"="Top I") -> ("Numeric"=w369:dbl)  [unwired: 9 in, 1 out]
              n209 = call-poly <vilib>:"NT Read Value.vi"("Name"="Bottom P") -> ("Numeric"=w382:dbl)  [unwired: 9 in, 1 out]
              n210 = call-poly <vilib>:"NT Read Value.vi"("Name"="Bottom I") -> ("Numeric"=w383:dbl)  [unwired: 9 in, 1 out]
              n211 = call-poly <vilib>:"NT Read Value.vi"("Name"="Top D") -> ("Numeric"=w370:dbl)  [unwired: 9 in, 1 out]
              n212 = call <vilib>:"WPI_CANTalonSRX_SetPID.vi"("CAN Talon SRX Ref"=w360, "P"=w368, "I"=w369, "D"=w370, "F"=0.0) -> ("CAN Talon SRX Ref"=w359:T8)  [unwired: 9 in, 1 out]
              n213 = call-poly <vilib>:"NT Read Value.vi"("Name"="Bottom D") -> ("Numeric"=w384:dbl)  [unwired: 9 in, 1 out]
              n214 = call <vilib>:"WPI_CANTalonSRX_SetPID.vi"("CAN Talon SRX Ref"=w373, "P"=w382, "I"=w383, "D"=w384, "F"=0.0) -> ("CAN Talon SRX Ref"=w377:T8)  [unwired: 9 in, 1 out]
              n215 = call <vilib>:"WPI_CANTalonSRX_ChangeMode.vi"("Output"=1.0, "Control Mode"=WPI_CANTalonSRX_APIControlMode."Percent VBus", "CAN Talon SRX Ref"=w359) -> ()  [unwired: 7 in, 2 out]
              n216 = call <vilib>:"WPI_CANTalonSRX_ChangeMode.vi"("Output"=0.0, "Control Mode"=WPI_CANTalonSRX_APIControlMode."Speed", "CAN Talon SRX Ref"=w377) -> ()  [unwired: 7 in, 2 out]
            }
            frame True {
              n217 = call <vilib>:"WPI_MotorControlRefNum Registry Get.vi"("refnum name"="Top Shooter") -> ("MotorControlDevRef"=w415:T8)  [unwired: 9 in, 1 out]
              n218 = call <vilib>:"WPI_MotorControlRefNum Registry Get.vi"("refnum name"="Bottom Shooter") -> ("MotorControlDevRef"=w401:T8)  [unwired: 9 in, 1 out]
              n219 = call <vilib>:"WPI_CANTalonSRX_SetReference.vi"("Reverse Closed-Loop Output"=TRUE, "Feedback Reference"=WPI_CANTalonSRX_APIFeedbackSelect."Count on Quad-A (Rising-Edge)", "CAN Talon SRX Ref"=w415) -> ("CAN Talon SRX Ref"=w416:T8)  [unwired: 7 in, 1 out]
              n220 = call <vilib>:"WPI_CANTalonSRX_SetReference.vi"("Feedback Reference"=WPI_CANTalonSRX_APIFeedbackSelect."Count on Quad-A (Rising-Edge)", "CAN Talon SRX Ref"=w401) -> ("CAN Talon SRX Ref"=w402:T8)  [unwired: 8 in, 1 out]
              n221 = call-poly <vilib>:"NT Read Value.vi"("Name"="Top P") -> ("Numeric"=w407:dbl)  [unwired: 9 in, 1 out]
              n222 = call-poly <vilib>:"NT Read Value.vi"("Name"="Top I") -> ("Numeric"=w406:dbl)  [unwired: 9 in, 1 out]
              n223 = call-poly <vilib>:"NT Read Value.vi"("Name"="Bottom P") -> ("Numeric"=w393:dbl)  [unwired: 9 in, 1 out]
              n224 = call-poly <vilib>:"NT Read Value.vi"("Name"="Bottom I") -> ("Numeric"=w392:dbl)  [unwired: 9 in, 1 out]
              n225 = call-poly <vilib>:"NT Read Value.vi"("Name"="Top D") -> ("Numeric"=w405:dbl)  [unwired: 9 in, 1 out]
              n226 = call <vilib>:"WPI_CANTalonSRX_SetPID.vi"("CAN Talon SRX Ref"=w416, "P"=w407, "I"=w406, "D"=w405, "F"=0.0) -> ("CAN Talon SRX Ref"=w412:T8)  [unwired: 9 in, 1 out]
              n227 = call-poly <vilib>:"NT Read Value.vi"("Name"="Bottom D") -> ("Numeric"=w391:dbl)  [unwired: 9 in, 1 out]
              n228 = call <vilib>:"WPI_CANTalonSRX_SetPID.vi"("CAN Talon SRX Ref"=w402, "P"=w393, "I"=w392, "D"=w391, "F"=0.0) -> ("CAN Talon SRX Ref"=w398:T8)  [unwired: 9 in, 1 out]
              n229 = call-poly <vilib>:"NT Read Value.vi"("Name"="Top Speed") -> ("Numeric"=w388:dbl)  [unwired: 9 in, 1 out]
              n230 = call <vilib>:"WPI_CANTalonSRX_ChangeMode.vi"("Output"=w388, "Control Mode"=WPI_CANTalonSRX_APIControlMode."Speed", "CAN Talon SRX Ref"=w412) -> ()  [unwired: 7 in, 2 out]
              n231 = call-poly <vilib>:"NT Read Value.vi"("Name"="Bottom Speed") -> ("Numeric"=w386:dbl)  [unwired: 9 in, 1 out]
              n232 = call <vilib>:"WPI_CANTalonSRX_ChangeMode.vi"("Output"=w386, "Control Mode"=WPI_CANTalonSRX_APIControlMode."Speed", "CAN Talon SRX Ref"=w398) -> ()  [unwired: 7 in, 2 out]
            }
          }
        }
      }
    }
  }
  n233 = disable-structure shown="Disabled" {
    frame Disabled {
      n234 = Absolute Value() -> (x=w422:dbl, abs(x)=w425:dbl)
      n235 = Greater?(x=w425, y=0.1) -> (0:w426:bool)
      n236 = Select(t=w422, s=w426, f=0.0) -> (s? t:f=w418:dbl)
      n237 = call <vilib>:"WPI_MotorControlRefNum Registry Get.vi"("refnum name"="Talon 1") -> ("MotorControlDevRef"=w428:T8)  [unwired: 9 in, 1 out]
      n238 = call <vilib>:"WPI_MotorControlSetOutput.vi"("Output"=w418, "MotorControlDevRef"=w428) -> ()  [unwired: 7 in, 3 out]
      n239 = call <vilib>:"WPI_MotorControlRefNum Registry Get.vi"("refnum name"="Talon 2") -> ("MotorControlDevRef"=w421:T8)  [unwired: 9 in, 1 out]
      n240 = call <vilib>:"WPI_MotorControlSetOutput.vi"("Output"=w418, "MotorControlDevRef"=w421) -> ()  [unwired: 7 in, 3 out]
      n241 = call <vilib>:"WPI_MotorControlRefNum Registry Get.vi"("refnum name"="Talon 3") -> ("MotorControlDevRef"=w419:T8)  [unwired: 9 in, 1 out]
      n242 = call <vilib>:"WPI_MotorControlSetOutput.vi"("Output"=w418, "MotorControlDevRef"=w419) -> ()  [unwired: 7 in, 3 out]
    }
    frame Enabled {
    }
  }
  n243 = disable-structure shown="Disabled" {
    disable-tunnel: _ -> [w429 _]
    frame Disabled {
      n244 = feedback #1() -> (w442:dbl)  [unwired: 1 in]
      n245 = feedback #2() -> (w438:dbl)  [unwired: 1 in]
      n246 = feedback #3() -> (w447:bool)  [unwired: 1 in]
      n247 = feedback #4() -> (w435:dbl)  [unwired: 1 in]
      n248 = call <vilib>:"SD Read Boolean.vi"("Name"="speed mode") -> ("Boolean"=w446:bool)  [unwired: 8 in, 2 out]
      n249 = feedback-in #3(w446) -> ()
      n250 = call <vilib>:"SD Read Number.vi"("Name"="P") -> ("Numeric"=w441:dbl)  [unwired: 8 in, 2 out]
      n251 = feedback-in #1(w441) -> ()
      n252 = call <vilib>:"SD Read Number.vi"("Name"="I") -> ("Numeric"=w437:dbl)  [unwired: 8 in, 2 out]
      n253 = feedback-in #2(w437) -> ()
      n254 = call <vilib>:"SD Read Number.vi"("Name"="D") -> ("Numeric"=w434:dbl)  [unwired: 8 in, 2 out]
      n255 = feedback-in #4(w434) -> ()
      n256 = Equal?(x=w441, y=w442) -> (x = y?=w440:bool)
      n257 = Equal?(x=w438, y=w437) -> (x = y?=w436:bool)
      n258 = Equal?(x=w446, y=w447) -> (x = y?=w439:bool)
      n259 = Equal?(x=w435, y=w434) -> (x = y?=w433:bool)
      n260 = And(x=w439, y=w440) -> (x .and. y?=w431:bool)
      n261 = And(x=w436, y=w433) -> (x .and. y?=w432:bool)
      n262 = Not And(1:w432, 2:w431) -> (0:w430:bool)
      n263 = case shown="False" w430 {
        tunnel: w446 -> [_ w463]
        tunnel: w441 -> [_ w462]
        tunnel: w437 -> [_ w461]
        tunnel: w434 -> [_ w460]
        tunnel: w429 -> [w449 _]
        frame False {
          n264 = call <vilib>:"SD Read Number.vi"("Name"="Shooter Speed" ("refnum name")) -> ("Numeric"=w453:dbl)  [unwired: 8 in, 2 out]
          n265 = case shown="True" w449 {
            tunnel: [0.0 ("Output") w459] -> w452
            tunnel: w453 -> [_ w459]
            frame False {
            }
            frame True {
            }
          }
          n266 = call <vilib>:"WPI_MotorControlRefNum Registry Get.vi"("refnum name"="shooterMotor") -> ("error out"=w457:errorcluster, "MotorControlDevRef"=w456:T8)  [unwired: 9 in]
          n267 = call <vilib>:"WPI_MotorControlSetOutput.vi"("error in (no error)"=w457, "Output"=w452, "MotorControlDevRef"=w456) -> ("Motor Output"=w454:dbl)  [unwired: 6 in, 2 out]
          n268 = call <vilib>:"SD Write Number.vi"("Numeric"=w454, "Name"="PID-JAG-VALUE") -> ()  [unwired: 8 in, 2 out]
        }
        frame True {
          n269 = case shown="True" w463 {
            tunnel: w462 -> [_ w479]
            tunnel: w461 -> [_ w470]
            tunnel: w460 -> [_ _]
            frame False {
              n270 = call-poly <vilib>:"WPI_MotorControlOpen.vi"("Device Number"=u8 44, "Control Mode"=WPI_CANJaguar_ControlMode."Percent VBus") -> ("error out"=w466:errorcluster, "MotorControlDeviceRef"=w467:T8)  [unwired: 8 in]
              n271 = call <vilib>:"WPI_MotorControlRefNum Registry Set.vi"("error in (no error)"=w466, "refnum name"="shooterMotor", "MotorControlDevRef"=w467) -> ()  [unwired: 7 in, 2 out]
            }
            frame True {
              w471 = T22 0 items=["Encoder"=0, "Inv Encoder"=2, "Quad Encoder"=3, "None"=255] ("Speed Reference")
              n272 = call-poly <vilib>:"WPI_MotorControlOpen.vi"("Device Number"=u8 44, "Control Mode"=WPI_CANTalonSRX_APIControlMode."Speed") -> ("error out"=w481:errorcluster, "MotorControlDeviceRef"=w478:T8)  [unwired: 8 in]
              n273 = call <vilib>:"WPI_CANTalonSRX_SetReference.vi"("error in (no error)"=w481, "Feedback Reference"=w471, "CAN Talon SRX Ref"=w478) -> ("error out"=w475:errorcluster, "CAN Talon SRX Ref"=w477:T8)  [unwired: 7 in]
              n274 = call <vilib>:"WPI_CANTalonSRX_ConfigEncoderCodesPerLine.vi"("CAN Talon SRX Ref"=w477, "Number Encoder Lines\n(Counts Per Rotation)"=u16 250 ("Encoder Codes Per Rev"), "error in (no error)"=w475) -> ("CAN Talon SRX Ref"=w476:T8, "error out"=w474:errorcluster)  [unwired: 11 in]
              n275 = call <vilib>:"WPI_CANTalonSRX_SetPID.vi"("CAN Talon SRX Ref"=w476, "P"=w479, "I"=w470, "error in (no error)"=w474) -> ("CAN Talon SRX Ref"=w472:T8, "error out"=w473:errorcluster)  [unwired: 10 in]
              n276 = call <vilib>:"WPI_MotorControlEnable.vi"("error in (no error)"=w473, "Encoder Initial Position"=0.0, "CAN MotorDevRef"=w472) -> ("error out"=w486:errorcluster, "CAN MotorDevRef"=w485:T8)  [unwired: 7 in]
              n277 = call <vilib>:"WPI_MotorControlRefNum Registry Set.vi"("error in (no error)"=w486, "refnum name"="shooterMotor", "MotorControlDevRef"=w485) -> ()  [unwired: 7 in, 2 out]
            }
          }
        }
      }
    }
    frame Enabled {
    }
  }
